vi "json_decode.vi"(8 "error in (no error)":errorcluster, 11 "json":string) -> (0 "error out":errorcluster, 3 "pairs":cluster{"key":string, "value":variant}[](array[cluster]))   [LabVIEW 2017]
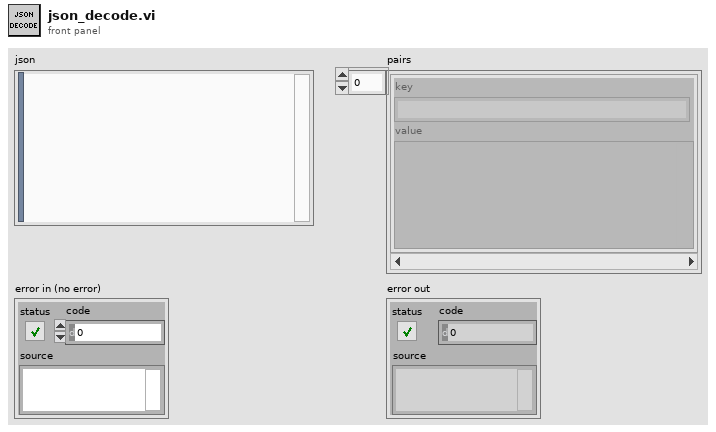
[diagram p1: front panel]
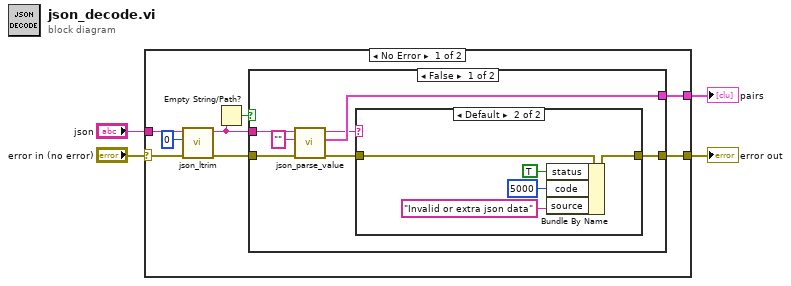
[diagram p0: block diagram]
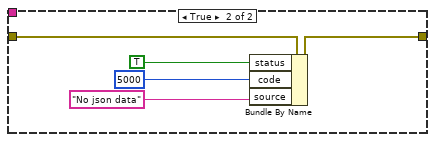
[diagram p3: hidden frame]
diagram:
  n1 = case shown="No Error" "error in (no error)" {
    selector: "error in (no error)" -> [w11 w30]
    tunnel: "json" -> [w7 _]
    tunnel: [w10 _] -> w2
    tunnel: [w9 w30] -> w1
    frame No Error {
      n2 = call "json_ltrim.vi"("offset (0)"=0, "data"=w7) -> ("left trim whitespace"=w6:string)  [unwired: 9 in]
      n3 = Empty String/Path?(string/path=w6) -> (empty?=w8:bool)
      n4 = case shown="False" w8 {
        tunnel: w11 -> [w18 w26]
        tunnel: w6 -> [w17 _]
        tunnel: [w15 _] -> w10
        tunnel: [w13 w25] -> w9
        frame False {
          n5 = call "json_parse_value.vi"("error in (no error)"=w18, "key"="", "data"=w17) -> ("error out"=w16:errorcluster, "pairs"=w15:cluster{"key":string, "value":variant}[], "remaining data"=w12:string)  [unwired: 6 in]
          n6 = case shown="Default" w12 {
            tunnel: w16 -> [w19 w24]
            tunnel: [w19 w23] -> w13
            frame "" {
            }
            frame Default {
              n7 = Bundle By Name(cluster=w24, "status"=TRUE, "code"=5000, "source"="Invalid or extra json data") -> (w23:errorcluster)
            }
          }
        }
        frame True {
          n8 = Bundle By Name(cluster=w26, "status"=TRUE, "code"=5000, "source"="No json data") -> (w25:errorcluster)
        }
      }
    }
    frame Error {
    }
  }
  "error out" <- w1
  "pairs" <- w2
